vi "Set Sessions DC Power.vi"(11 "Semiconductor Module Context":T1) -> (0 "error out":errorcluster, 1 "Channel Ids":string[](array[string]), 2 "Instrument Names":string[](array[string]))   [LabVIEW 2013]
uses:
  <vilib>/NI_TestStand_SemiconductorModule/NI_TestStand_Semiconductor_Module.lvlibp/PinMap/General/SemiconductorModuleContext.ctl
  <vilib>/NI_TestStand_SemiconductorModule/NI_TestStand_Semiconductor_Module.lvlibp
panel:
  out "Instrument Handle Array":refnum<k15>[](array[refnum])
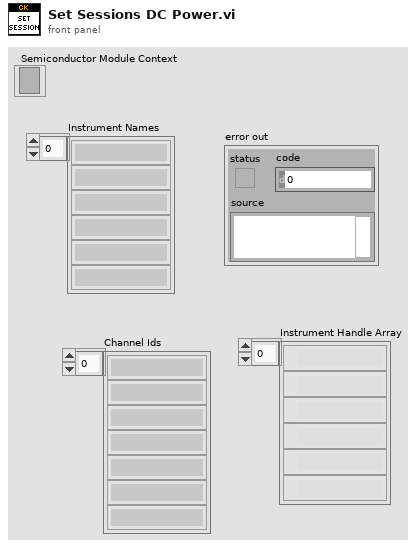
[diagram p1: front panel]
types:
  T1 = typedef "NI_TestStand_Semiconductor_Module.lvlibp/SemiconductorModuleContext.ctl" = refnum<k7>
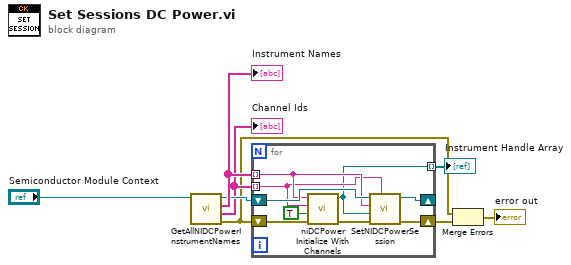
[diagram p0: block diagram]
diagram:
  n1 = call <vilib>:"GetAllNIDCPowerInstrumentNames.vi"("Semiconductor Module Context"="Semiconductor Module Context") -> ("error out"=w3:errorcluster, "Channel Ids"=w6:string[], "Instrument Names"=w8:string[], "Semiconductor Module Context Out"=w7:T1)  [unwired: 7 in]
  "Instrument Names" <- w8
  "Channel Ids" <- w6
  n2 = for {
    tunnel: w8 -> [w13] mode=indexing
    shift-right: [w16] -> _
    shift-left: w7 -> [w17]
    shift-right: [w15] -> w2
    shift-left: w3 -> [w14]
    tunnel: w6 -> [w11] mode=indexing
    tunnel: [w9] -> w1 mode=indexing
    n3 = call <instrlib>:"niDCPower Initialize With Channels.vi"("error in (no error)"=w14, "reset (false)"=TRUE, "channels"=w11, "resource name"=w13) -> ("error out"=w12:errorcluster, "instrument handle out"=w9:refnum<k15>)  [unwired: 6 in]
    n4 = call <vilib>:"SetNIDCPowerSession.vi"("Channel Id"=w11, "error in (no error)"=w12, "Instrument Session"=w9, "Instrument Name"=w13, "Semiconductor Module Context"=w17) -> ("error out"=w15:errorcluster, "Semiconductor Module Context Out"=w16:T1)  [unwired: 5 in]
  }
  "Instrument Handle Array" <- w1
  n5 = Merge Errors(w3, w2) -> (→"error out":errorcluster)
